vi "23384_Davis_Poku_Amankwa_Amankwa.DavisPoku.MNE1201.8.5c_348265_547221251.vi"() -> ()   [LabVIEW 2018]
panel:
  in  "Number of Elements":i32
  out "While Loop Time (ms)":u32
  out "While Loop Array":i32[](array[numeric])
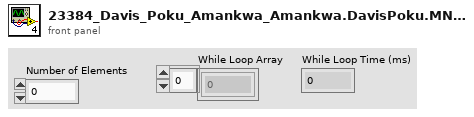
[diagram p1: front panel]
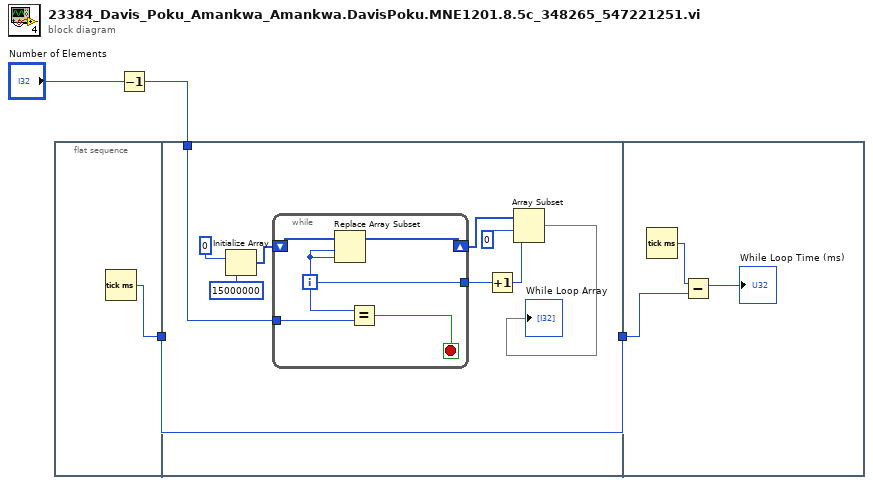
[diagram p0: block diagram]
diagram:
  n1 = flat-sequence {
    tunnel: [w5] -> w4
    tunnel: w1 -> [w12]
    tunnel: w4 -> [w14]
    tunnel: [w14] -> w3
    tunnel: w3 -> [w21]
    frame #0 {
      n2 = Tick Count (ms)() -> (millisecond timer value=w5:u32)
    }
    frame #1 {
      n3 = Initialize Array(0, 15000000) -> (w11:i32[])
      n4 = while {
        shift-right: [w19] -> w10
        shift-left: w11 -> [w20]
        tunnel: w12 -> [w17]
        tunnel: [w16] -> w8
        i -> [w16]
        stop <- w18 stop-if-true
        n5 = Replace Array Subset(array=w20, new element=w16, index=w16) -> (w19:i32[])
        n6 = Equal?(x=w16, y=w17) -> (x = y?=w18:bool)
      }
      n7 = Increment(x=w8) -> (x+1=w7:i32)
      n8 = Array Subset(array=w10, index=0, length=w7) -> (→"While Loop Array":i32[])
    }
    frame #2 {
      n9 = Tick Count (ms)() -> (millisecond timer value=w23:u32)
      n10 = Subtract(x=w23, y=w21) -> (x-y=→"While Loop Time (ms)":u32)
    }
  }
  n11 = Decrement(x="Number of Elements") -> (x-1=w1:i32)
